vi "Get State.vi"(8 "error in (no error)":errorcluster, 11 "Connection in":refnum<class "Connection.lvclass">) -> (0 "error out":errorcluster, 2 "State":T1, 3 "Connection out":refnum<class "Connection.lvclass">)   [LabVIEW 2020, in "Stream.lvlib" / "Connection.lvclass"]
doc: "Returns the current state of the connection as one of the following values:\n\n<b>Closed</b> - The instance has been closed and is no longer usable.\n\n<b>Idle</b> - The instance is ready to be used and <b>Open</b> can be called to establish the connection.\n\n<b>Connecting</b> - The connection is currently in the process of establishing the connection. This may be the case when trying to open the network connection or initializing some resource.\n\n<b>Connected</b> - The connection has been establish and the <b>Stream</b> can be retrieved to start reading and writing data.\n\n<b>Shutdown</b> - The instance is currently in the process of closing down and can no longer be used. After shutdown has completed, the state should change to \"Closed\"."
uses:
  Connection.lvclass
  State.ctl
  Connection.lvclass/Connection.ctl
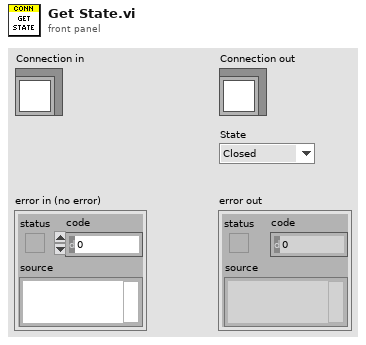
[diagram p1: front panel]
types:
  T1 = typedef "Stream.lvlib/Connection.lvclass/State.ctl" = enum16{"Closed", "Idle", "Connecting", "Connected", "Shutdown"}
  T2 = typedef "Stream.lvlib/Connection.lvclass/Ref Data.ctl" = cluster{"State":T1}
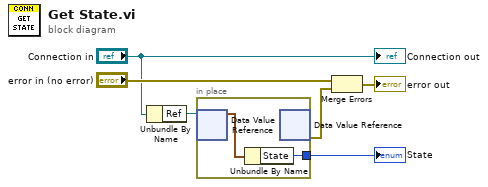
[diagram p0: block diagram]
diagram:
  n1 = Unbundle By Name("Connection in") -> ("Ref"=w5:refnum<data-value>)
  n2 = in-place {
    in-place-border: [w7] -> w3
    n3 = in-place-dvr #1(w5) -> (w8:T2)  [unwired: 1 out]
    n4 = Unbundle By Name(w8) -> ("State"=w7:T1)
    n5 = in-place-dvr #1() -> (w1:errorcluster)  [unwired: 1 in, 1 out]
  }
  "State" <- w3
  n6 = Merge Errors("error in (no error)", w1) -> (→"error out":errorcluster)
  "Connection out" <- "Connection in"
